vi "ToRepo.vi"(8 "error in":errorcluster, 9 "to repo cluster":T1, 10 "repository in":refnum<class "NISE_CEF_Repository.lvclass">, 11 "node in":refnum<class "module editor node.lvclass">) -> (0 "error out":errorcluster, 2 "repository out":refnum<class "NISE_CEF_Repository.lvclass">, 3 "node out":refnum<class "module editor node.lvclass">)   [LabVIEW 2013, in "PL Framework Configuration Tool.lvlib" / "module editor node.lvclass"]
doc: "Transfers the information from the tree node into the repo. How it is stored in the repo depends on the Repo."
uses:
  module editor node.lvclass
  <vilib>/CEF_TreeControl/Repository/NISE_CEF_Repository.lvclass
  <vilib>/CEF_TreeControl/Node/ToRepoCluster.ctl
  to repo data.ctl
  SystemConfigRepo/SystemConfigRepo.lvclass
  SystemConfigRepo/SystemConfigRepo.lvclass/SystemConfigRepo.ctl
  TBM Configuration Node/TBM Configuration Node.lvclass
  <vilib>/NI/Tag Bus Module Framework/root configuration/set metadata property.vi
  <vilib>/CEF_TreeControl/Node/NISE_CEF_Node.lvclass
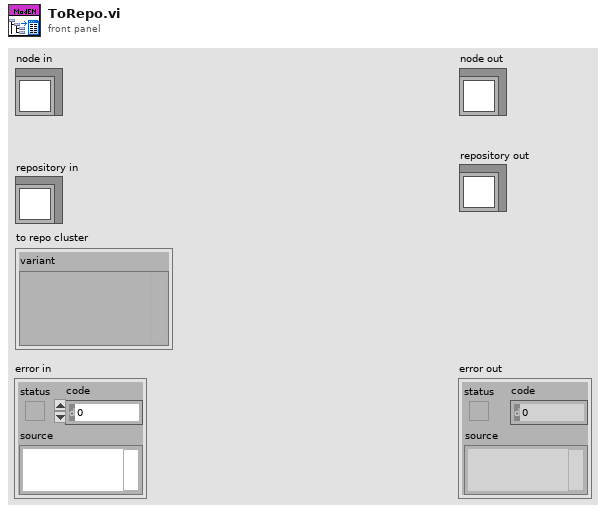
[diagram p1: front panel]
types:
  T1 = typedef "NISE_CEF_Node.lvclass/ToRepoCluster.ctl" = cluster{"variant":variant}
  T2 = typedef "PL Framework Configuration Tool.lvlib/module editor node.lvclass/to repo data.ctl" = cluster{"target index":i32, "engine index":i32}
  T3 = typedef "PLConfigurationSerializer.lvlib/targets cluster.ctl" = cluster{"Target Configuration":refnum<class "PL_Target Configuration.lvclass">, "engines":T4[]}
  T4 = typedef "PLConfigurationSerializer.lvlib/engines cluster.ctl" = cluster{"engine configuration":refnum<class "engine configuration.lvclass">, "modules":refnum<class "TBM module configuration.lvclass">[]}
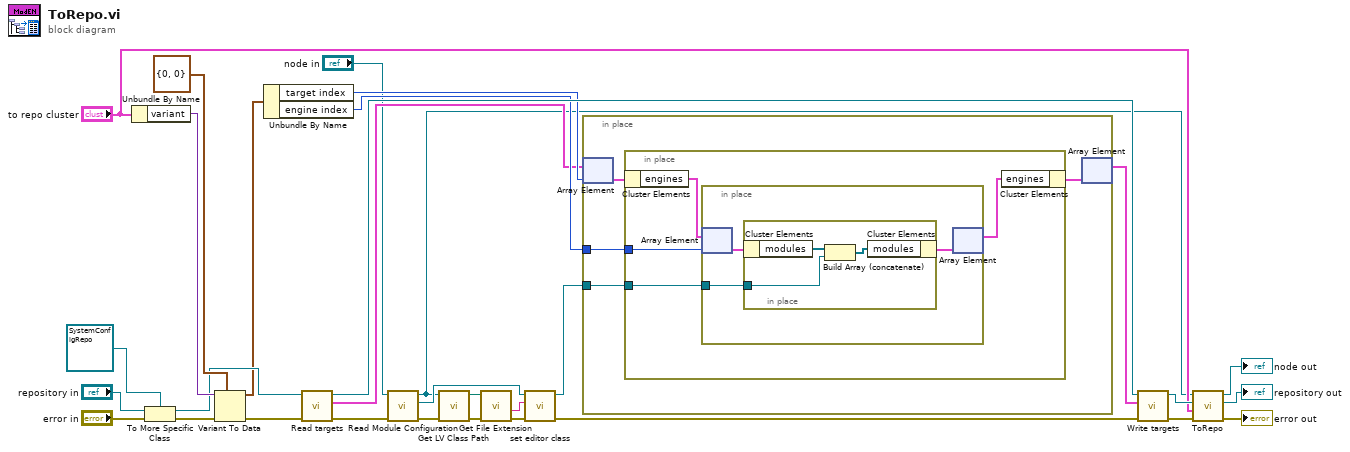
[diagram p0: block diagram]
diagram:
  n1 = Unbundle By Name("to repo cluster") -> ("variant"=w27:variant)
  n2 = To More Specific Class(target class=refnum<class "SystemConfigRepo.lvclass"> refnum ("SystemConfigRepo.lvclass"), reference="repository in", error in="error in") -> (specific class reference=w25:refnum<class "SystemConfigRepo.lvclass">, error out=w28:errorcluster)
  n3 = Variant To Data(error in=w28, type=T2 {"target index"=0, "engine index"=0} ("to repo data"), Variant=w27) -> (data=w23:T2, error out=w13:errorcluster)
  n4 = Unbundle By Name(w23) -> ("target index"=w22:i32, "engine index"=w21:i32)
  n5 = call "Read targets.vi"("error in"=w13, "SystemConfigRepo in"=w25) -> ("error out"=w10:errorcluster, "targets"=w14:T3[], "SystemConfigRepo out"=w24:refnum<class "SystemConfigRepo.lvclass">)  [unwired: 7 in]
  n6 = call "Read Module Configuration.vi"("error in"=w10, "Module Editor Node in"="node in") -> ("error out"=w2:errorcluster, "module configuration"=w11:refnum<class "TBM module configuration.lvclass">, "Module Editor Node out"=w1:refnum<class "module editor node.lvclass">)  [unwired: 7 in]
  n7 = call <vilib>:"Get LV Class Path.vi"("error in (no error)"=w2, "object"=w1) -> ("error out"=w7:errorcluster, "class path"=w5:path)  [unwired: 8 in]
  n8 = call <vilib>:"Get File Extension.vi"("error in (no error)"=w7, "file"=w5) -> ("error out"=w6:errorcluster, "filename without extension"=w4:string)  [unwired: 6 in, 2 out]
  n9 = call "set editor class.vi"("error in"=w6, "editor class"=w4, "configuration in"=w11) -> ("error out"=w8:errorcluster, "configuration out"=w9:refnum<class "TBM module configuration.lvclass">)  [unwired: 7 in]
  n10 = in-place {
    in-place-border: w21 -> [w33]
    in-place-border: w9 -> [w32]
    n11 = in-place-array #1(w14, w22) -> (w35:T3)
    n12 = in-place {
      in-place-border: w33 -> [w37]
      in-place-border: w32 -> [w36]
      n13 = in-place-cluster #2(w35) -> ("engines"=w39:T4[])
      n14 = in-place {
        in-place-border: w36 -> [w40]
        n15 = in-place-array #3(w39, w37) -> (w41:T4)
        n16 = in-place {
          in-place-border: w40 -> [w43]
          n17 = in-place-cluster #4(w41) -> ("modules"=w45:refnum<class "TBM module configuration.lvclass">[])
          n18 = Build Array (concatenate)(w45, w43) -> (w44:refnum<class "TBM module configuration.lvclass">[])
          n19 = in-place-cluster #4("modules"=w44) -> (w42:T4)
        }
        n20 = in-place-array #3(w42) -> (w38:T4[])  [unwired: 1 out]
      }
      n21 = in-place-cluster #2("engines"=w38) -> (w34:T3)
    }
    n22 = in-place-array #1(w34) -> (w12:T3[])  [unwired: 1 out]
  }
  n23 = call "Write targets.vi"("error in"=w8, "targets"=w12, "SystemConfigRepo in"=w24) -> ("error out"=w19:errorcluster, "SystemConfigRepo out"=w18:refnum<class "SystemConfigRepo.lvclass">)  [unwired: 7 in]
  n24 = call-parent "ToRepo.vi"("error in"=w19, "to repo cluster"="to repo cluster", "repository in"=w18, "node in"=w1) -> ("error out"=→"error out":errorcluster, "repository out"=→"repository out":refnum<class "NISE_CEF_Repository.lvclass">, "node out"=→"node out":refnum<class "module editor node.lvclass">)  [unwired: 5 in]
